vi "Trav_pos_for_Email.vi"() -> (0 "String":string)   [LabVIEW 2010]
uses:
  Controls/Overhead.ctl
  Globals/Trav_pos_global.vi
  Globals/Meas_global.vi
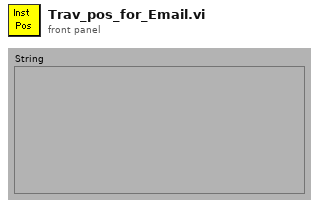
[diagram p1: front panel]
types:
  T1 = typedef "Overhead.ctl" = enum16{"Update total times", "Read Current Overhead", "Re Scale totals to 3 hrs", "Initialise totals to 3hr"}
  T2 = typedef "Tunnel_Coordinates.ctl" = enum16{"Work in Tunnel Coordinates", "Work in Model Coordinates"}
  T3 = typedef "Traverse_cluster.ctl" = cluster{"Start X":dbl, "Start Y":dbl, "Start Z":dbl, "End X":dbl, "End Y":dbl, "End Z":dbl, "No. of pts.":i32, "Spacing":T4, "Filename":path, "Tunnel Speed":dbl, "Averaging time (min)":dbl, "Extra Commands":string, "Specific Arguments":string, "Emission Rate (l/min)":dbl, "Trace Gas Concentration (%)":dbl, "Density Ratio":string, "Comments":string, "Row No":i32, "Row Type Selector":T5, "Completion time":string, "Row Duration (mins)":dbl, "No. of Valid pts.":i32, "Meas Setup File":string}
  T4 = typedef "Spacing.ctl" = enum16{"Linear", "Log", "Gauss", "Specified", "N/A"}
  T5 = typedef "Multi_run_mode.ctl" = enum16{"Move Traverse Only", "Set Tunnel Speed Only", "Set Source Only", "Set Measurement Conditions", "Single Measurement", "Vertical Profile", "Lateral Profile", "Longitudinal Profile", "Explore Volume", "Multi-Axis Profile", "Auto Calibrate", "Meas Fast FID Bkgnd", "Check Beam Power", "Scanning Valve Measurement", "Run VI Named:", "Set ADAM Ch", "Wait (minutes)", "Send Message", "Synchronize With:", "Fall Back to this Row", "Turn Off Row Repeating", "Blank Row"}
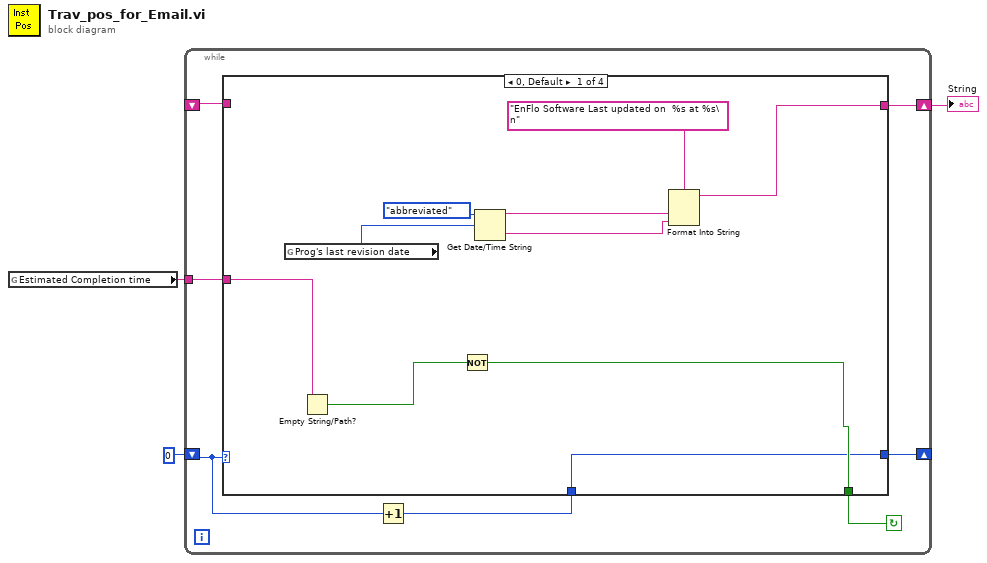
[diagram p0: block diagram]
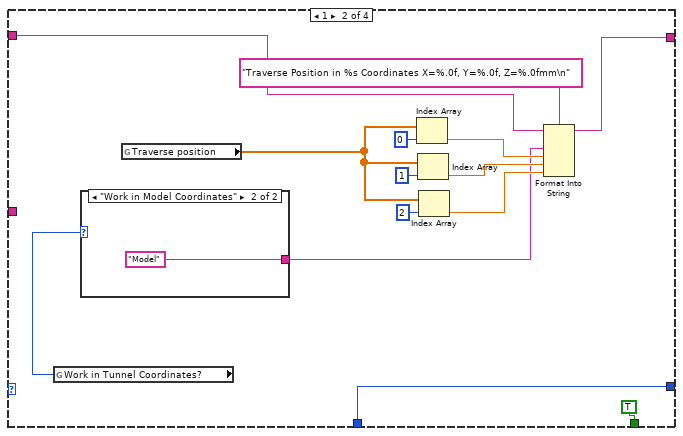
[diagram p2: hidden frame]
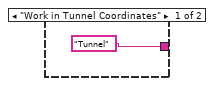
[diagram p3: hidden frame]
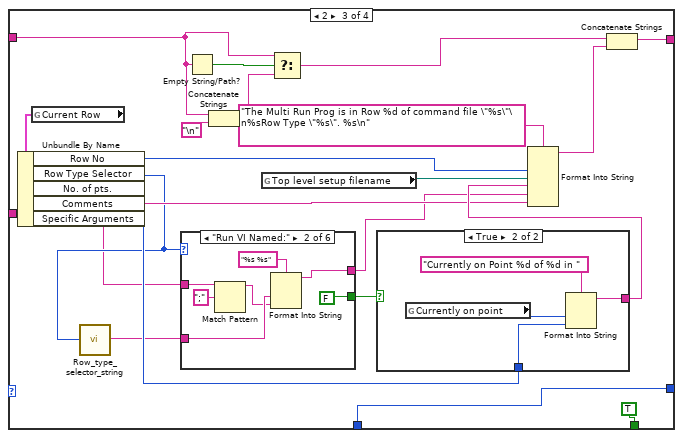
[diagram p4: hidden frame]
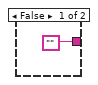
[diagram p5: hidden frame]
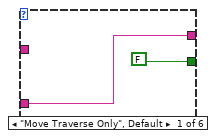
[diagram p6: hidden frame]
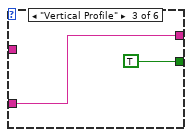
[diagram p7: hidden frame]
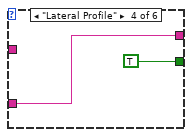
[diagram p8: hidden frame]
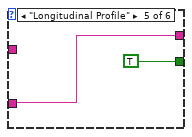
[diagram p9: hidden frame]
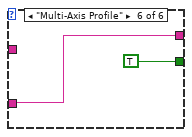
[diagram p10: hidden frame]
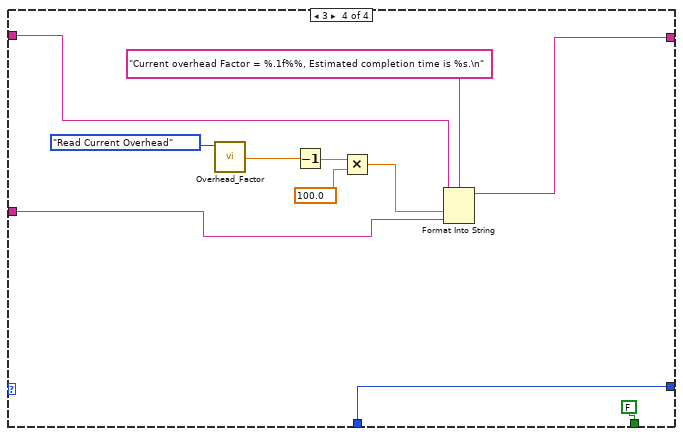
[diagram p11: hidden frame]
diagram:
  n1 = global read "Trav_pos_global.vi" "Estimated Completion time"() -> (w1:string)
  n2 = while {
    shift-left: _ -> [w5]
    shift-right: [w7] -> w2
    shift-left: 0 -> [w10]
    shift-right: [w9] -> _
    tunnel: w1 -> [w4]
    stop <- w6 continue-if-true
    n3 = Increment(x=w10) -> (x+1=w8:i32)
    n4 = case shown="0, Default" w10 {
      tunnel: [w17 w34 w51 w89] -> w9
      tunnel: w8 -> [w17 w34 w51 w89]
      tunnel: [w11 w25 w57 w81] -> w7
      tunnel: [w18 TRUE TRUE FALSE] -> w6
      tunnel: w5 -> [_ w26 w48 w82]
      tunnel: w4 -> [w20 _ _ w80]
      frame 0, Default {
        n5 = global read "Meas_global.vi" "Prog's last revision date"() -> (w15:u32)
        n6 = Empty String/Path?(string/path=w20) -> (empty?=w19:bool)
        n7 = Not(x=w19) -> (.not. x?=w18:bool)
        n8 = Get Date/Time String(date format (0)=enum16{"short", "long", "abbreviated"}."abbreviated", seconds (now)=w15) -> (date string=w13:string, time string=w12:string)  [unwired: 1 out]
        n9 = Format Into String(format string="EnFlo Software Last updated on  %s at %s\n" ("Format String"), w13, w12) -> (resulting string=w11:string)  [unwired: 2 in, 1 out]
      }
      frame 1 {
        n10 = global read "Trav_pos_global.vi" "Work in Tunnel Coordinates?"() -> (w24:T2)
        n11 = case shown="\"Work in Model Coordinates\"" w24 {
          tunnel: ["Tunnel" "Model"] -> w22
          frame "Work in Tunnel Coordinates" {
          }
          frame "Work in Model Coordinates" {
          }
        }
        n12 = global read "Trav_pos_global.vi" "Traverse position"() -> (w21:dbl[])
        n13 = Index Array(array=w21, index=0) -> (element=w23:dbl)
        n14 = Index Array(array=w21, index=1) -> (element=w28:dbl)
        n15 = Index Array(array=w21, index=2) -> (element=w27:dbl)
        n16 = Format Into String(format string="Traverse Position in %s Coordinates X=%.0f, Y=%.0f, Z=%.0fmm\n" ("Format String"), initial string=w26, w22, w23, w28, w27) -> (resulting string=w25:string)  [unwired: 1 in, 1 out]
      }
      frame 2 {
        n17 = global read "Trav_pos_global.vi" "Current Row"() -> (w42:T3)
        n18 = Unbundle By Name(w42) -> ("Row No"=w56:i32, "Row Type Selector"=w40:T5, "No. of pts."=w54:i32, "Comments"=w41:string, "Specific Arguments"=w37:string)
        n19 = call "Row_type_selector_string.vi"("Mode"=w40) -> ("Output string"=w39:string)
        n20 = case shown="\"Run VI Named:\"" w40 {
          tunnel: [FALSE FALSE TRUE TRUE TRUE TRUE] -> w55
          tunnel: w39 -> [w63 w70 w72 w74 w76 w78]
          tunnel: [w63 w68 w72 w74 w76 w78] -> w38
          tunnel: w37 -> [_ w66 _ _ _ _]
          frame "Move Traverse Only", Default {
          }
          frame "Run VI Named:" {
            n21 = Match Pattern(string=w66, regular expression=";") -> (before substring=w65:string)  [unwired: 4 out]
            n22 = Format Into String(format string="%s %s" ("Format String"), w70, w65) -> (resulting string=w68:string)  [unwired: 2 in, 1 out]
          }
          frame "Vertical Profile" {
          }
          frame "Lateral Profile" {
          }
          frame "Longitudinal Profile" {
          }
          frame "Multi-Axis Profile" {
          }
        }
        n23 = Empty String/Path?(string/path=w48) -> (empty?=w50:bool)
        n24 = Concatenate Strings(w48, "\n") -> (w49:string)
        n25 = global read "Trav_pos_global.vi" "Top level setup filename"() -> (w45:path)
        n26 = Select(t=w48, s=w50, f=w49) -> (s? t:f=w47:string)
        n27 = case shown="True" w55 {
          tunnel: w54 -> [_ w61]
          tunnel: ["" w59] -> w44
          frame False {
          }
          frame True {
            n28 = global read "Trav_pos_global.vi" "Currently on point"() -> (w62:i32)
            n29 = Format Into String(format string="Currently on Point %d of %d in " ("Format String"), w62, w61) -> (resulting string=w59:string)  [unwired: 2 in, 1 out]
          }
        }
        n30 = Format Into String(format string="The Multi Run Prog is in Row %d of command file \"%s\"\n%sRow Type \"%s\". %s\n" ("Format String"), w56, w45, w44, w38, w41) -> (resulting string=w43:string)  [unwired: 2 in, 1 out]
        n31 = Concatenate Strings(w47, w43) -> (w57:string)
      }
      frame 3 {
        n32 = call "Overhead_Factor.vi"("Mode"=Overhead."Read Current Overhead") -> ("Current Overhead Factor"=w87:dbl)  [unwired: 3 in]
        n33 = Decrement(x=w87) -> (x-1=w86:dbl)
        n34 = Multiply(x=w86, y=100.0) -> (x*y=w84:dbl)
        n35 = Format Into String(format string="Current overhead Factor = %.1f%%, Estimated completion time is %s.\n" ("Format String"), initial string=w82, w84, w80) -> (resulting string=w81:string)  [unwired: 1 in, 1 out]
      }
    }
  }
  "String" <- w2
